vi "Chirp.vi"(6 "icfft":i32, 9 "Chirp FFT Pairs":T1[](array[typedef]), 10 "Sub-band Sample Rate":dbl, 11 "binWorkUnitDataPoints.bin (DataIn) in":csg[](array[numeric])) -> (0 "d":sgl=-0.01266181, 1 "c":sgl=0.99991983, 2 "binWorkUnitDataPoints.bin (DataIn) out":csg[](array[numeric]), 3 "Chirp/Fft Pair 1 - Fft Length":i32, 4 "ang":dbl=1.9979847564988014, 5 "time":dbl=26.84345694384995, 7 "Chirp/Fft Pair 1 - Chirp Rate":dbl)   [LabVIEW 2015, in "SETI_LV.lvlib"]
uses:
  SETI_LV.lvlib
  TypeDefs/ChirpFFT Pairs.ctl
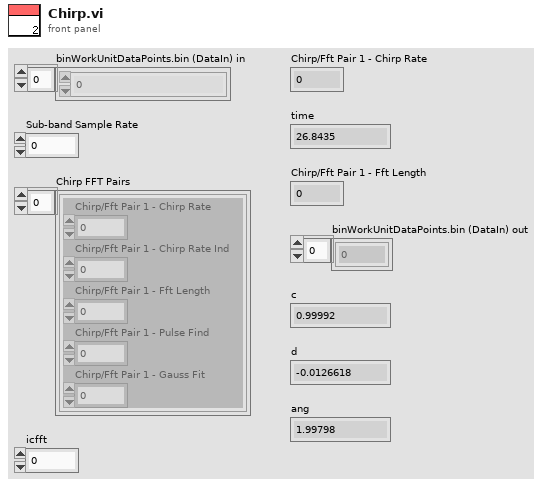
[diagram p1: front panel]
types:
  T1 = typedef "SETI_LV.lvlib/ChirpFFT Pairs.ctl" = cluster{"Chirp/Fft Pair 1 - Chirp Rate":dbl, "Chirp/Fft Pair 1 - Chirp Rate Ind":i32, "Chirp/Fft Pair 1 - Fft Length":i32, "Chirp/Fft Pair 1 - Pulse Find":i32, "Chirp/Fft Pair 1 - Gauss Fit":i32}
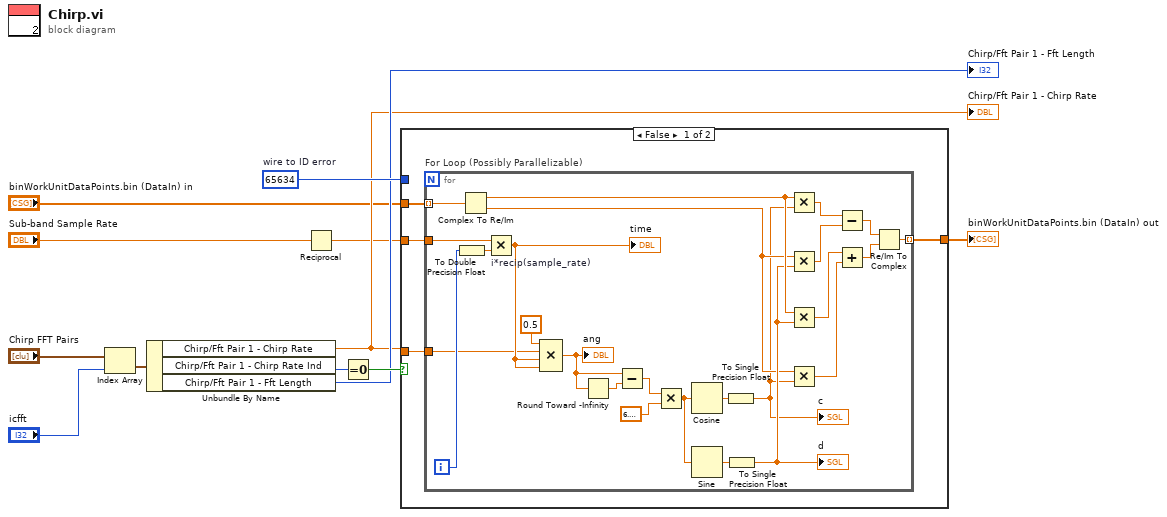
[diagram p0: block diagram]
diagram:
  w11 = 65634  # wire to ID error
  n1 = Index Array(array="Chirp FFT Pairs", index="icfft") -> (element=w2:T1)
  n2 = Unbundle By Name(w2) -> ("Chirp/Fft Pair 1 - Chirp Rate"=w7:dbl, "Chirp/Fft Pair 1 - Chirp Rate Ind"=w3:i32, "Chirp/Fft Pair 1 - Fft Length"=→"Chirp/Fft Pair 1 - Fft Length":i32)
  "Chirp/Fft Pair 1 - Chirp Rate" <- w7
  n3 = Reciprocal(x="Sub-band Sample Rate") -> (1/x=w6:dbl)
  n4 = Equal To 0?(x=w3) -> (x = 0?=w10:bool)
  n5 = case shown="False" w10 {
    tunnel: "binWorkUnitDataPoints.bin (DataIn) in" -> [w16 w42]
    tunnel: [w13 w42] -> w8
    tunnel: w6 -> [w15 _]
    tunnel: w7 -> [w14 _]
    tunnel: w11 -> [_ _]
    frame False {
      n6 = for "For Loop (Possibly Parallelizable)" {
        tunnel: w16 -> [w41] mode=indexing
        tunnel: w15 -> [w40]
        tunnel: w14 -> [w35]
        tunnel: [w18] -> w13 mode=indexing
        i -> [w39]
        n7 = To Double Precision Float(number=w39) -> (double precision float=w38:dbl)
        n8 = Complex To Re/Im(x + iy=w41) -> (x=w22:sgl, y=w20:sgl)
        n9 = Multiply "i*recip(sample_rate)"(x=w40, y=w38) -> (x*y=w37:dbl)
        "time" <- w37
        n10 = Compound Arithmetic op=MULTIPLY(0.5 ("value"), w35, w37, w37) -> (w34:dbl)
        "ang" <- w34
        n11 = Round Toward -Infinity(1:w34) -> (0:w33:dbl)
        n12 = Subtract(x=w34, y=w33) -> (x-y=w32:dbl)
        n13 = Multiply(x=w32, y=6.283185307179586) -> (x*y=w30:dbl)
        n14 = Cosine(x=w30) -> (cos(x)=w28:dbl)
        n15 = Sine(x=w30) -> (sin(x)=w29:dbl)
        n16 = To Single Precision Float(number=w28) -> (single precision float=w19:sgl)
        "c" <- w19
        n17 = To Single Precision Float(number=w29) -> (single precision float=w21:sgl)
        "d" <- w21
        n18 = Multiply(x=w22, y=w19) -> (x*y=w27:sgl)
        n19 = Multiply(x=w20, y=w21) -> (x*y=w26:sgl)
        n20 = Multiply(x=w22, y=w21) -> (x*y=w23:sgl)
        n21 = Multiply(x=w20, y=w19) -> (x*y=w24:sgl)
        n22 = Subtract(x=w27, y=w26) -> (x-y=w25:sgl)
        n23 = Add(x=w23, y=w24) -> (x+y=w17:sgl)
        n24 = Re/Im To Complex(1:w17, 2:w25) -> (0:w18:csg)
      }
    }
    frame True {
    }
  }
  "binWorkUnitDataPoints.bin (DataIn) out" <- w8
